vi "PR Tags.vi"(11 "PR Module Configs":T1[](array[typedef]) {"Settings"."PID 2 Parameters"."output range"."output low" format="%.2f"; "Settings"."PID 2 Parameters"."output range"."output high" min=0.0 max=100.0 format="%.2f"; "Settings"."PID 2 Parameters"."PID gains"."derivative time (Td, min)" format="%.3f"; "Settings"."PID 2 Parameters"."PID gains"."integral time (Ti, min)" format="%.3f"; "Settings"."PID 2 Parameters"."PID gains"."proportional gain (Kc)" format="%.3f"}) -> (1 "PID 2 Out Tag 2":string, 2 "All  Numeric Tags 6":string[](array[string]), 3 "All Boolean Tags 6":string[](array[string]), 4 "PR Module Tags Array":T6[](array[typedef]), 5 "4-20mA Module Tag Names":T6)   [LabVIEW 2018]
uses:
  Pressure Regulator Control Module/Pressure Regulator/Controls/4-20mA Module Tag Names Cluster.ctl
  Pressure Regulator Control Module/Pressure Regulator/Controls/4-20mA Module Config Cluster.ctl
  <vilib>/Utility/miscctls.llb/LVPoint32TypeDef.ctl
  Pressure Regulator Control Module/Pressure Regulator/Controls/4-20mA Module Settings Cluster.ctl
  Pressure Transmitter/Pressure Transmitter Device Settings.ctl
  Pressure Reg Module/Pressure Regulator Device Settings.ctl
  Pressure Regulator Control Module/Pressure Regulator/4-20mA Module.lvlib
  Pressure Transmitter/Pressure Transmitter Library.lvlib
  Pressure Reg Module/Pressure Regulator Library.lvlib
panel:
  # "Instrument Settings"
  # "Instrument Settings"
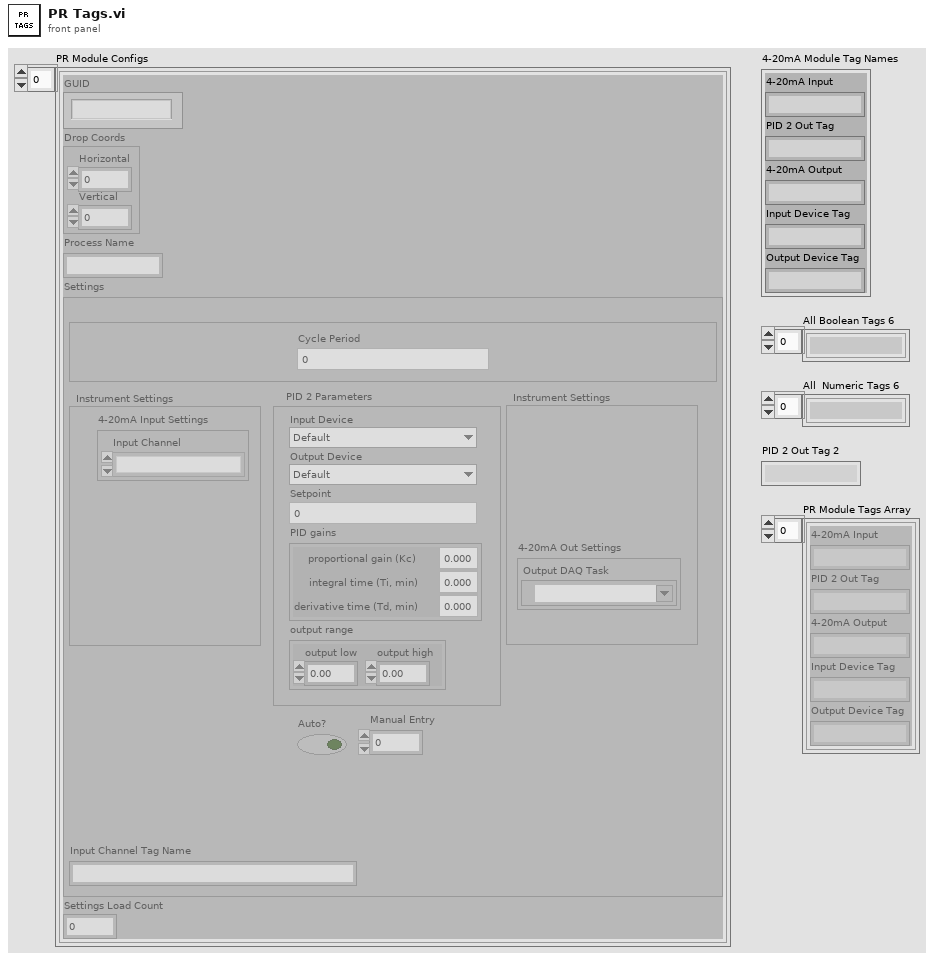
[diagram p1: front panel]
types:
  T1 = typedef "4-20mA Module.lvlib/4-20mA Module Config Cluster.ctl" = cluster{"GUID":string, "Drop Coords":T2, "Process Name":string, "Settings":T3, "Settings Load Count":i32}
  T2 = typedef "LVPoint32TypeDef.ctl" = cluster{"Horizontal":i32, "Vertical":i32}
  T3 = typedef "4-20mA Module.lvlib/4-20mA Module Settings Cluster.ctl" = cluster{"Cycle Period":dbl, "PID 2 Parameters":cluster{"Input Device":enum16{"Default", "4-20mA"}, "Output Device":enum16{"Default", "Equilibar Pressure Reg", "Flow Regulator"}, "Setpoint":dbl, "PID gains":cluster{"proportional gain (Kc)":dbl, "integral time (Ti, min)":dbl, "derivative time (Td, min)":dbl}, "output range":cluster{"output low":dbl, "output high":dbl}}, "Manual Entry":dbl, "Auto?":bool, "4-20mA Input Settings":T4, "4-20mA Out Settings":T5, "Input Channel Tag Name ":string}
  T4 = typedef "Pressure Transmitter Library.lvlib/Pressure Transmitter Device Settings.ctl" = cluster{"Input Channel ":u16}
  T5 = typedef "Pressure Regulator Library.lvlib/Pressure Regulator Device Settings.ctl" = cluster{"Output DAQ Task":refnum<k21>}
  T6 = typedef "4-20mA Module.lvlib/4-20mA Module Tag Names Cluster.ctl" = cluster{"4-20mA Input":string, "PID 2 Out Tag":string, "4-20mA Output":string, "Input Device Tag":string, "Output Device Tag":string}
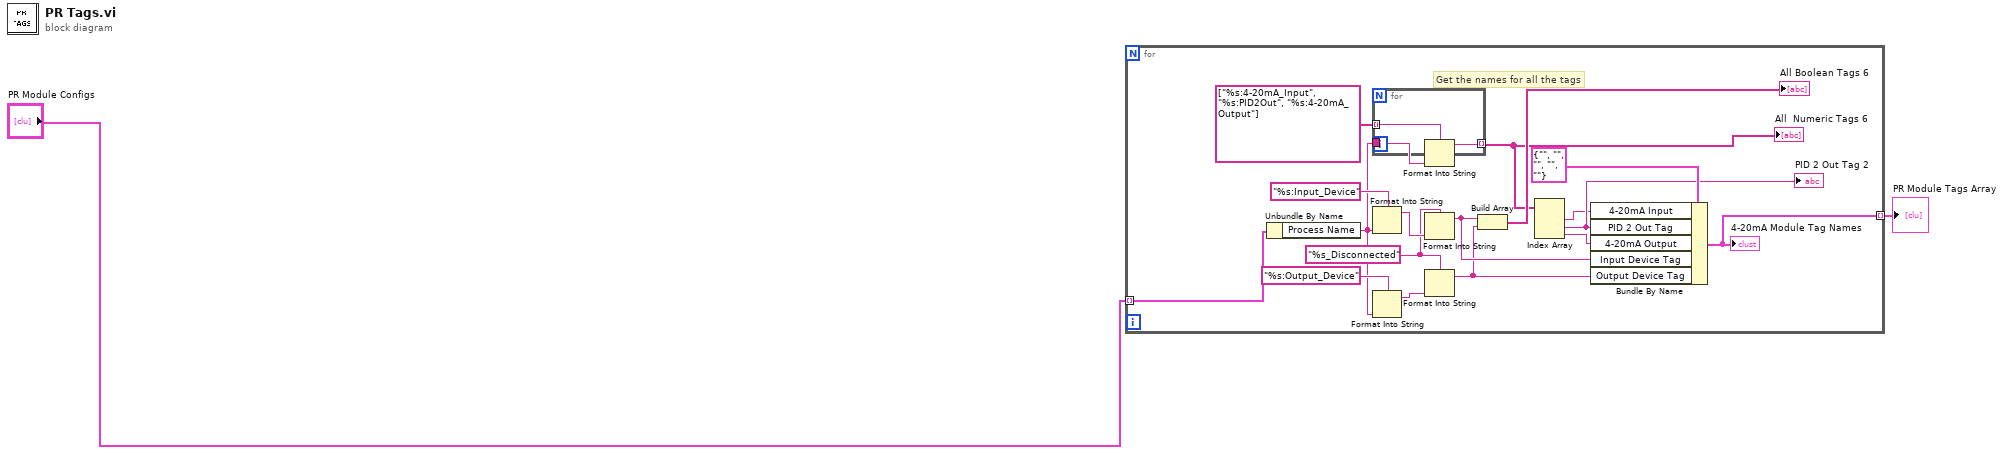
[diagram p0: block diagram]
diagram:
  n1 = for {
    tunnel: "PR Module Configs" -> [w4] mode=indexing
    tunnel: [w3] -> w2 mode=indexing
    w5 = "%s_Disconnected"
    # "Get the names for all the tags"
    n2 = Unbundle By Name(w4) -> ("Process Name"=w10:string)
    n3 = for {
      tunnel: string[] ["%s:4-20mA_Input", "%s:PID2Out", "%s:4-20mA_Output"] -> [w22] mode=indexing
      tunnel: w10 -> [w21]
      tunnel: [w20] -> w9 mode=indexing
      n4 = Format Into String(format string=w22, w21) -> (resulting string=w20:string)  [unwired: 2 in, 1 out]
    }
    "All  Numeric Tags 6" <- w9
    n5 = Format Into String(format string="%s:Input_Device", w10) -> (resulting string=w18:string)  [unwired: 2 in, 1 out]
    n6 = Format Into String(format string="%s:Output_Device", w10) -> (resulting string=w17:string)  [unwired: 2 in, 1 out]
    n7 = Format Into String(format string=w5, w18) -> (resulting string=w12:string)  [unwired: 2 in, 1 out]
    n8 = Format Into String(format string=w5, w17) -> (resulting string=w11:string)  [unwired: 2 in, 1 out]
    n9 = Build Array(w12, w11) -> (→"All Boolean Tags 6":string[])
    n10 = Index Array(array=w9) -> (element #1=w7:string, element #2=w8:string, element #3=w6:string)  [unwired: 3 in]
    "PID 2 Out Tag 2" <- w8
    n11 = Bundle By Name(cluster=T6 {"4-20mA Input"="", "PID 2 Out Tag"="", "4-20mA Output"="", "Input Device Tag"="", "Output Device Tag"=""} ("Feed Module Tag Names"), "4-20mA Input"=w7, "PID 2 Out Tag"=w8, "4-20mA Output"=w6, "Input Device Tag"=w12, "Output Device Tag"=w11) -> (w3:T6)
    "4-20mA Module Tag Names" <- w3
  }
  "PR Module Tags Array" <- w2
